vi "CU_test_NeuralNet.vi"(6 "DataTypes":T1=enum."Test Data", 8 "error in":errorcluster, 9 "ANN in":T2={"Training Data"={"dim in"=0, "dim out"=0, "# samples"=0, "Input"=[], "Output"=[]}, "Normalize Info"={"input min"=[], "input max"=[], "output min"=[], "output max"=[]}, "3-layer NN"={"# input neuron "=0, "# hidden neuron"=0, "# output neuron"=0, "Weight (I->H)"=[], "Weight (H->O)"=[], "Output"=[], "Hidden Out"=[], "Derivation Output"=[], "Derivation Hidden"=[], "dw (I->H)"=[], "dw (H->O)"=[]}, "Ternimal Condition"={"min MSE"=1e-05, "min delta MSE"=1e-05, "min step length"=1e-08, "max iteration"=inf}}, 10 "Indices":i8[](array[numeric]), 11 "ClassifierClass in":refnum<class "ClassifierClass.lvclass">) -> (0 "error out":errorcluster, 1 "Accuracy":dbl, 2 "Confusion Matrix":i32[][](array[numeric]), 3 "ClassifierClass out":refnum<class "ClassifierClass.lvclass">)   [LabVIEW 2016, in "Classifier.lvlib" / "ClassifierClass.lvclass"]
uses:
  ClassifierClass.lvclass
  <vilib>/addons/Machine Learning/Supervised Learning/ml_BP_Project.ctl
  <vilib>/addons/Machine Learning/Supervised Learning/ml_BP_Data.ctl
  <vilib>/addons/Machine Learning/Supervised Learning/ml_BP_Normalize Data.ctl
  <vilib>/addons/Machine Learning/Supervised Learning/ml_BP_3layer Feedforward.ctl
  <vilib>/addons/Machine Learning/Supervised Learning/ml_BP_Terminal Condition.ctl
  CU_DataTypes.ctl
  ClassifierClass.lvclass/ClassifierClass.ctl
  CU_CohenKappa.vi
  <vilib>/addons/Machine Learning/NILabs_MLT.lvlib
  Classifier.lvlib
panel:
  # "This VI is a part of BCI Design library, http://www.ru-bci.org \nCopyright © 2020, Sotnikov Peter, All rights reserved. License: CC BY-NC 4.0"
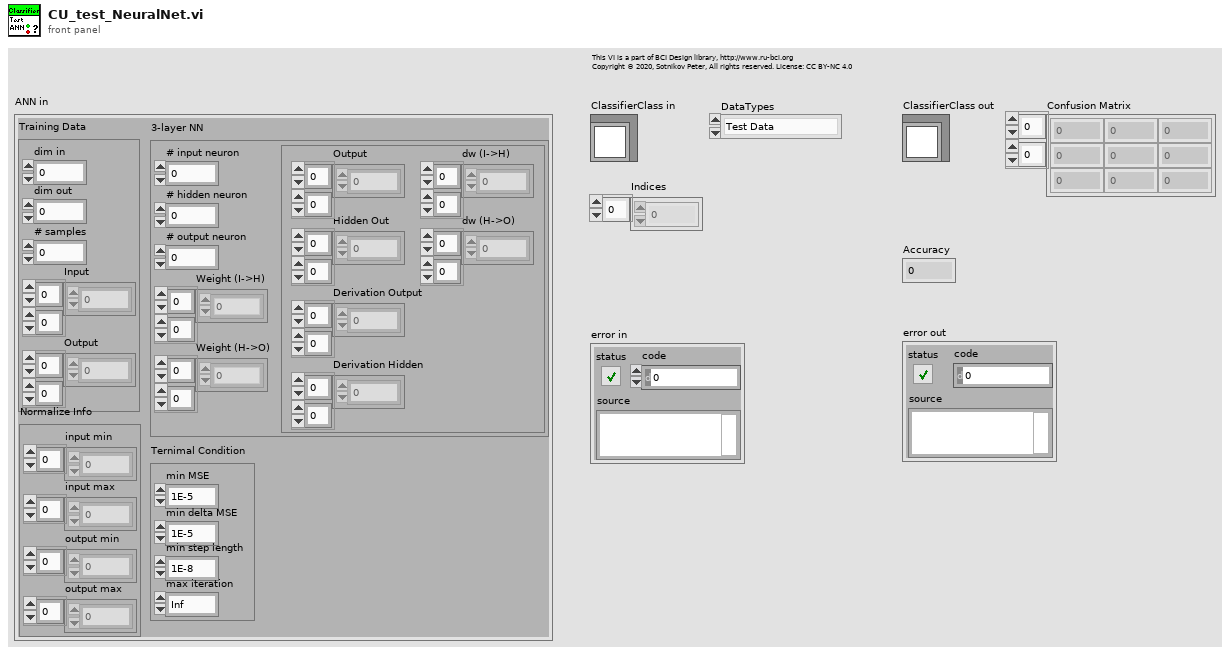
[diagram p1: front panel]
types:
  T1 = typedef "Classifier.lvlib/CU_DataTypes.ctl" = enum16{"Training Data", "Test Data", "Training Data (cross-check)", "Test Data (cross-check)"}
  T2 = typedef "NILabs_MLT.lvlib/ml_BP_Project.ctl" = cluster{"Training Data":T3, "Normalize Info":T4, "3-layer NN":T5, "Ternimal Condition":T6}
  T3 = typedef "NILabs_MLT.lvlib/ml_BP_Data.ctl" = cluster{"dim in":i32, "dim out":i32, "# samples":i32, "Input":dbl[][], "Output":dbl[][]}
  T4 = typedef "NILabs_MLT.lvlib/ml_BP_Normalize Data.ctl" = cluster{"input min":dbl[], "input max":dbl[], "output min":dbl[], "output max":dbl[]}
  T5 = typedef "NILabs_MLT.lvlib/ml_BP_3layer Feedforward.ctl" = cluster{"# input neuron ":i32, "# hidden neuron":i32, "# output neuron":i32, "Weight (I->H)":dbl[][], "Weight (H->O)":dbl[][], "Output":dbl[][], "Hidden Out":dbl[][], "Derivation Output":dbl[][], "Derivation Hidden":dbl[][], "dw (I->H)":dbl[][], "dw (H->O)":dbl[][]}
  T6 = typedef "NILabs_MLT.lvlib/ml_BP_Terminal Condition.ctl" = cluster{"min MSE":dbl, "min delta MSE":dbl, "min step length":dbl, "max iteration":dbl}
  T7 = typedef "XML_EEG_Features.lvlib/XML_FF_Trial.ctl" = cluster{"ClassLabel":string, "FeatureVector":dbl[]}
  T8 = typedef "Classifier.lvlib/CU_ClassifierQualityMeasure.ctl" = enum16{"Accuracy", "Cohen's kappa"}
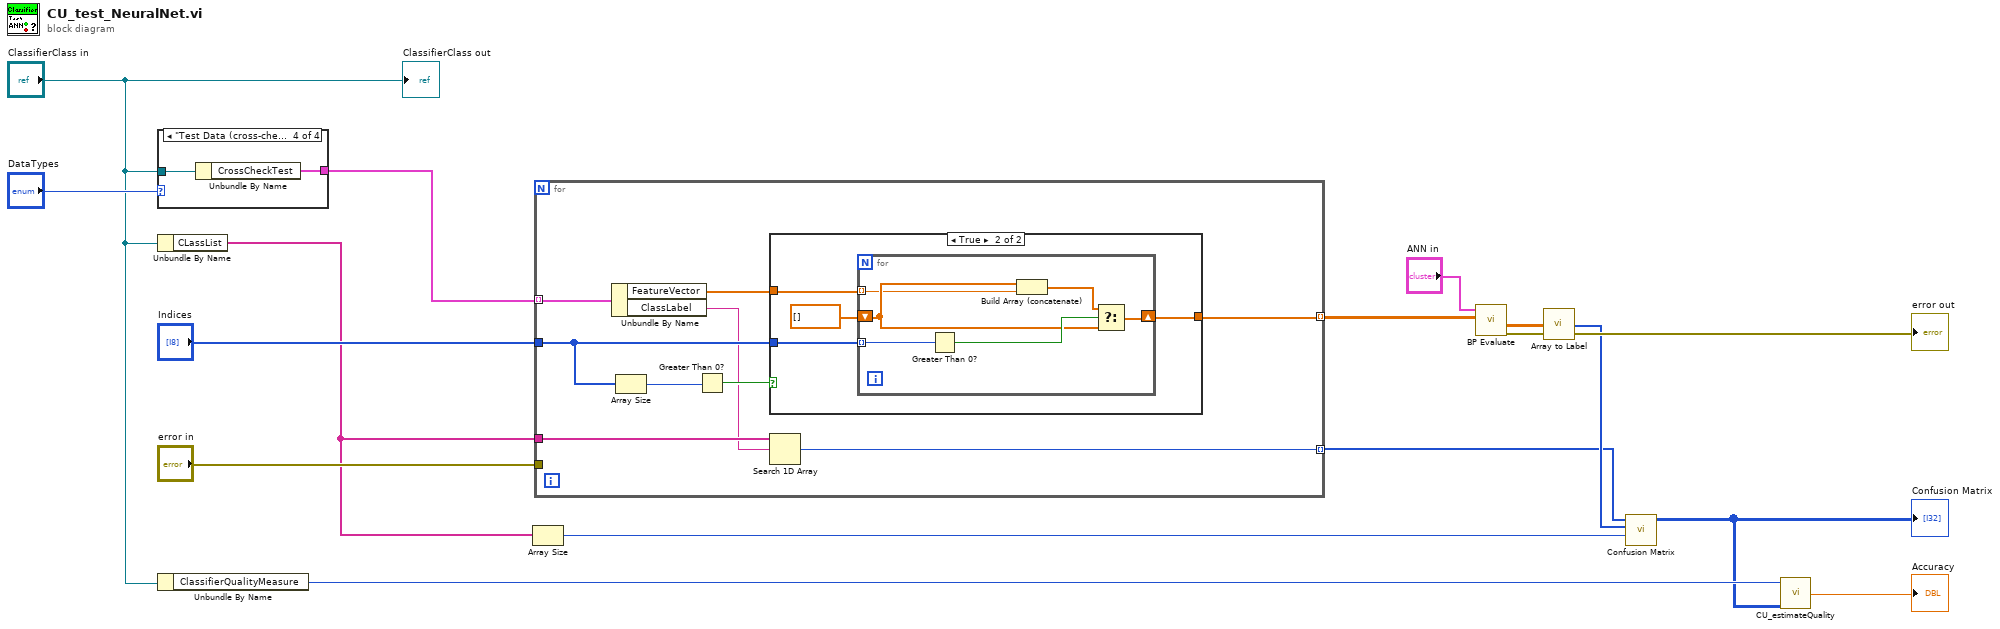
[diagram p0: block diagram]
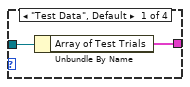
[diagram p2: hidden frame]
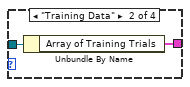
[diagram p3: hidden frame]
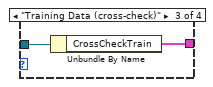
[diagram p4: hidden frame]
diagram:
  n1 = case shown="\"Test Data (cross-check)\"" "DataTypes" {
    tunnel: "ClassifierClass in" -> [w18 w20 w22 w24]
    tunnel: [w17 w19 w21 w23] -> w8
    frame "Test Data", Default {
      n2 = Unbundle By Name(w18) -> ("Array of Test Trials"=w17:T7[])
    }
    frame "Training Data" {
      n3 = Unbundle By Name(w20) -> ("Array of Training Trials"=w19:T7[])
    }
    frame "Training Data (cross-check)" {
      n4 = Unbundle By Name(w22) -> ("CrossCheckTrain"=w21:T7[])
    }
    frame "Test Data (cross-check)" {
      n5 = Unbundle By Name(w24) -> ("CrossCheckTest"=w23:T7[])
    }
  }
  n6 = Unbundle By Name("ClassifierClass in") -> ("CLassList"=w7:string[])
  n7 = Unbundle By Name("ClassifierClass in") -> ("ClassifierQualityMeasure"=w3:T8)
  n8 = Array Size(array=w7) -> (size(s)=w10:i32)
  n9 = for {
    tunnel: w8 -> [w31] mode=indexing
    tunnel: "Indices" -> [w29]
    tunnel: "error in" -> [_]
    tunnel: w7 -> [w28]
    tunnel: [w26] -> w13 mode=indexing
    tunnel: [w25] -> w4 mode=indexing
    n10 = Unbundle By Name(w31) -> ("FeatureVector"=w30:dbl[], "ClassLabel"=w27:string)
    n11 = Array Size(array=w29) -> (size(s)=w33:i32)
    n12 = Greater Than 0?(x=w33) -> (x > 0?=w32:bool)
    n13 = case shown="True" w32 {
      tunnel: w30 -> [w34 w38]
      tunnel: w29 -> [_ w37]
      tunnel: [w34 w35] -> w26
      frame False {
      }
      frame True {
        n14 = for {
          tunnel: w38 -> [w40] mode=indexing
          tunnel: w37 -> [w44] mode=indexing
          shift-right: [w43] -> w35
          shift-left: dbl[] [] -> [w41]
          n15 = Greater Than 0?(x=w44) -> (x > 0?=w42:bool)
          n16 = Build Array (concatenate)(w41, w40) -> (w39:dbl[])
          n17 = Select(t=w39, s=w42, f=w41) -> (s? t:f=w43:dbl[])
        }
      }
    }
    n18 = Search 1D Array(1D array=w28, element=w27) -> (index of element=w25:i32)  [unwired: 1 in]
  }
  n19 = call <vilib>:"BP Evaluate.vi"("Test data samples"=w13, "BP Project"="ANN in") -> ("error out"=→"error out":errorcluster, "NN outputs"=w11:dbl[][])  [unwired: 5 in, 3 out]
  n20 = call <vilib>:"Array to Label.vi"("Array"=w11) -> ("Classes"=w5:i32[])
  n21 = call <vilib>:"Confusion Matrix.vi"("# of classes"=w10, "Predicted class labels"=w5, "Actual class labels"=w4) -> ("Confusion Matrix"=w2:i32[][])  [unwired: 7 in, 1 out]
  "Confusion Matrix" <- w2
  n22 = call "CU_estimateQuality.vi"("Quality Measure in"=w3, "Confusion Matrix in"=w2) -> ("Classification Quality out"=→"Accuracy":dbl)  [unwired: 6 in]
  "ClassifierClass out" <- "ClassifierClass in"
